vi "Teleop.vi"(10 "Match Info":T1={"Autonomous Elapsed Seconds"=0.0, "TeleOp Elapsed Seconds"=0.0, "Disabled Elapsed Seconds"=0.0, "Visited Autonomous"=FALSE, "Visited TeleOp"=FALSE, "Visited Disabled"=FALSE, "Autonomous Settings"={"Autonomous Style"=enum."Independent", "VI Refnum"=refnum}}, 11 "Call Context":T2) -> ()   [LabVIEW 2015]
doc: "This VI is called for each TeleOp packet received from the DS where the robot is not disabled. It is often used to read from the joysticks and update I/O or to update setpoints for timed control loops. It should complete and return within 20 milliseconds or it may miss DS packets."
uses:
  <vilib>/Rock Robotics/WPI/DriverStation/WPI_DriverStationDerivedRobotMode.ctl
  <vilib>/Rock Robotics/WPI/DriverStation/WPI_DriverStationMatch Info.ctl
  <vilib>/Rock Robotics/WPI/Utilities/WPI_GetSetVariantRefNum.vi
  <vilib>/Rock Robotics/Network Tables/SD Write Numeric Array.vi
  <vilib>/Rock Robotics/Network Tables/SD Write Boolean Array.vi
  Robot Global Data.vi
  <vilib>/Rock Robotics/WPI/RobotDrive/WPI_RobotDriveMecanumDrive_Cartesian.vi
  SimpleGyro/SimpleGyro.lvlib
panel:
  out "Angle":dbl
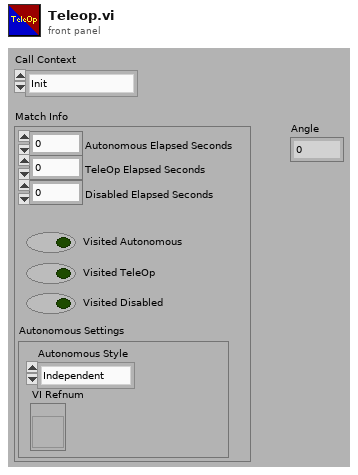
[diagram p1: front panel]
types:
  T1 = typedef "WPI_DriverStationMatch Info.ctl" = cluster{"Autonomous Elapsed Seconds":dbl, "TeleOp Elapsed Seconds":dbl, "Disabled Elapsed Seconds":dbl, "Visited Autonomous":bool, "Visited TeleOp":bool, "Visited Disabled":bool, "Autonomous Settings":cluster{"Autonomous Style":enum16{"Iterative", "Independent"}, "VI Refnum":refnum<vi>}}
  T2 = typedef "WPI_DriverStationDerivedRobotMode.ctl" = enum16{"Init", "Execute", "Stop"}
  T3 = typedef "WPI_JoystickDevRef.ctl" = cluster{"Device":T4}
  T4 = typedef "WPI_JoystickDeviceEnum.ctl" = enum16{"USB 0", "USB 1", "USB 2", "USB 3", "USB 4", "USB 5"}
  T5 = typedef "WPI_RobotDriveDevRef.ctl" = cluster{"DevStatus":errorcluster, "Motors[]":T6[], "Square Inputs":bool, "Max Output":dbl}
  T6 = typedef "WPI_MotorControlDeviceRef.ctl" = cluster{"DeviceStatus":errorcluster, "Type":T7, "PWM":cluster{"PWM Channel":T8, "DeadBand":T9}, "CAN":cluster{"Device Number":u8, "Control Mode":T10, "Semaphore":T11, "Max Vout":dbl, "TalonSRX Control Mode":T12}, "Invert":bool, "TransformRef":T13, "InvTransformRef":T13}
  T7 = typedef "WPI_MotorControlType.ctl" = enum16{"PWM", "CAN", "CANTalonSRX"}
  T8 = typedef "FPGA_DIOPWMChannel.ctl" = enum8{"PWM 0", "PWM 1", "PWM 2", "PWM 3", "PWM 4", "PWM 5", "PWM 6", "PWM 7", "PWM 8", "PWM 9", "PWM MXP 0", "PWM MXP 1", "PWM MXP 2", "PWM MXP 3", "PWM MXP 4", "PWM MXP 5", "PWM MXP 6", "PWM MXP 7", "PWM MXP 8", "PWM MXP 9", "Invalid"}
  T9 = typedef "WPI_PWMDeadband.ctl" = cluster{"Name":string, "maxPositivePwm":i32, "minPositivePwm":i32, "centerPwm":i32, "maxNegativePwm":i32, "minNegativePwm":i32, "angularRange":u16}
  T10 = typedef "WPI_CANJaguar_ControlMode.ctl" = enum8{"Percent VBus", "Current", "Speed", "Position", "Voltage"}
  T11 = typedef "Semaphore RefNum" = refnum<k1>
  T12 = typedef "WPI_CANTalonSRX_APIControlMode.ctl" = enum8{"Percent VBus", "Speed", "Position", "Slave", "Unchanged / Invalid"}
  T13 = typedef "WPI_PWMTransform_ConPane.ctl" = refnum<vi>
  T14 = typedef "SimpleGyro.lvlib/WPI_SimpleGyroDevRef.ctl" = cluster{"DevStatus":errorcluster, "Handle":i32, "SPI Bus":T15, "Device Found":bool, "Sample Rate":dbl}
  T15 = typedef "spi_bus.ctl" = enum16{"SPI On-Board, CS0", "SPI On-Board, CS1", "SPI On-Board, CS2", "SPI On-Board, CS3", "SPI MXP", "Invalid"}
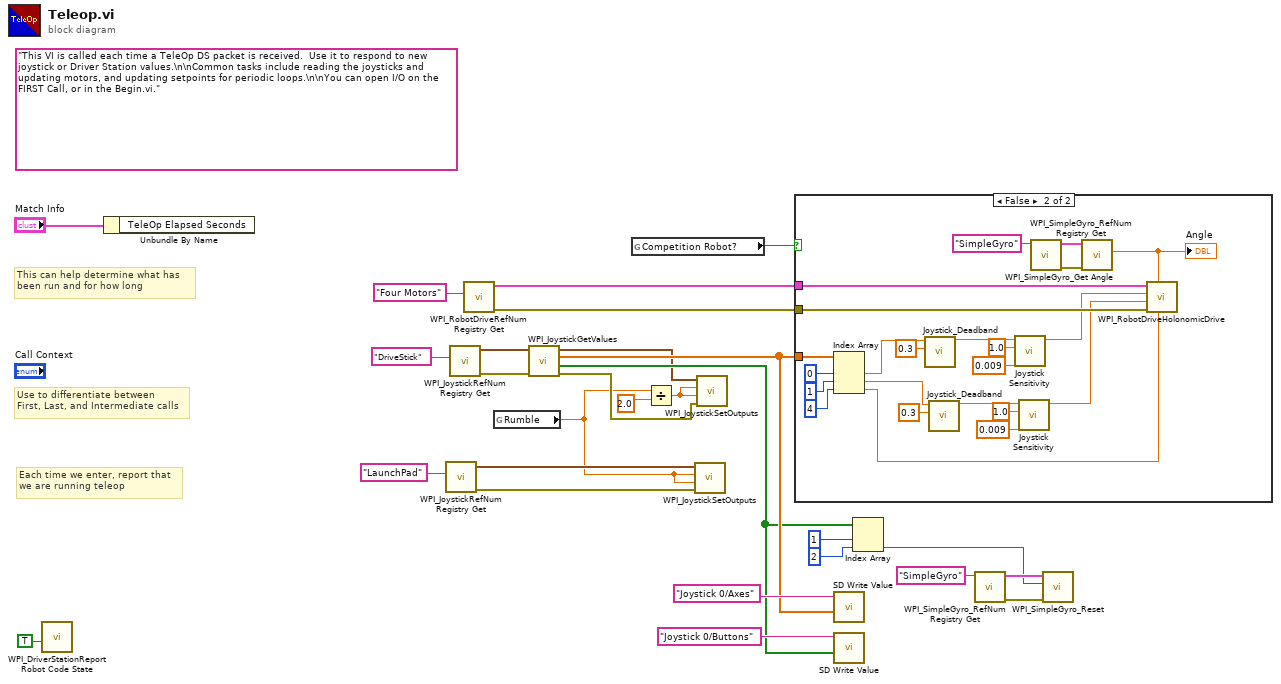
[diagram p0: block diagram]
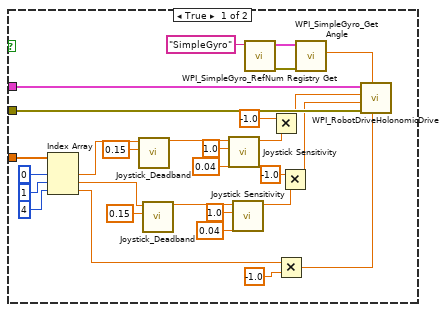
[diagram p2: hidden frame]
diagram:
  (unwired) "This VI is called each time a TeleOp DS packet is received.  Use it to respond to new joystick or Driver Station values.\n\nCommon tasks include reading the joysticks and updating motors, and updating setpoints for periodic loops.\n\nYou can open I/O on the FIRST Call, or in the Begin.vi."
  # "Each time we enter, report that\nwe are running teleop"
  # "Use to differentiate between\nFirst, Last, and Intermediate calls"
  # "This can help determine what has\nbeen run and for how long"
  n1 = call <vilib>:"WPI_DriverStationReport Robot Code State.vi"("TeleOp"=TRUE ("Autonomous")) -> ()  [unwired: 10 in, 1 out]
  n2 = Unbundle By Name("Match Info") -> ()  [unwired: 1 out]
  n3 = call <vilib>:"WPI_JoystickRefNum Registry Get.vi"("refnum name"="LaunchPad") -> ("error out"=w8:errorcluster, "JoystickDevRef"=w7:T3)  [unwired: 9 in]
  n4 = call <vilib>:"WPI_JoystickRefNum Registry Get.vi"("refnum name"="DriveStick") -> ("error out"=w19:errorcluster, "JoystickDevRef"=w21:T3)  [unwired: 9 in]
  n5 = call <vilib>:"WPI_RobotDriveRefNum Registry Get.vi"("refnum name"="Four Motors") -> ("error out"=w20:errorcluster, "RobotDriveDevRef"=w17:T5)  [unwired: 1 in, 8 out]
  n6 = global read "Robot Global Data.vi" "Rumble"() -> (w2:dbl)
  n7 = call <vilib>:"WPI_JoystickGetValues.vi"("error in (no error)"=w19, "JoystickDevRef"=w21) -> ("error out"=w10:errorcluster, "Buttons"=w22:bool[], "Axes"=w23:dbl[], "JoystickDevRef"=w11:T3)  [unwired: 5 in, 1 out]
  n8 = global read "Robot Global Data.vi" "Competition Robot?"() -> (w1:bool)
  n9 = Divide(x=w2, y=2.0) -> (x/y=w12:dbl)
  n10 = call <vilib>:"WPI_JoystickSetOutputs.vi"("error in (no error)"=w8, "Right Rumble"=w2, "Left Rumble"=w2, "JoystickDevRef"=w7) -> ()  [unwired: 6 in, 2 out]
  n11 = call <vilib>:"WPI_JoystickSetOutputs.vi"("error in (no error)"=w10, "Right Rumble"=w12, "Left Rumble"=w12, "JoystickDevRef"=w11) -> ()  [unwired: 6 in, 2 out]
  n12 = case shown="False" w1 {
    tunnel: w23 -> [w56 w79]
    tunnel: w20 -> [w55 w78]
    tunnel: w17 -> [w51 w74]
    frame True {
      n13 = Index Array(array=w56, index #1=0 ("index"), index #2=1 ("index"), index #3=4 ("index")) -> (element #1=w38:dbl, element #2=w43:dbl, element #3=w36:dbl)
      n14 = call "Joystick_Deadband.vi"("band"=0.15, "in"=w38) -> ("out"=w41:dbl)  [unwired: 9 in]
      n15 = call "Joystick_Deadband.vi"("band"=0.15, "in"=w43) -> ("out"=w46:dbl)  [unwired: 9 in]
      n16 = call "Joystick Sensitivity.vi"("B"=0.04, "A"=1.0, "X"=w41) -> ("Y"=w33:dbl)  [unwired: 8 in]
      n17 = call "Joystick Sensitivity.vi"("B"=0.04, "A"=1.0, "X"=w46) -> ("Y"=w32:dbl)  [unwired: 8 in]
      n18 = call "WPI_SimpleGyro_RefNum Registry Get.vi"("refnum name"="SimpleGyro") -> ("error out"=w47:errorcluster, "SimpleGyroDevRef"=w49:T14)  [unwired: 9 in]
      n19 = Multiply(x=-1.0, y=w33) -> (x*y=w31:dbl)
      n20 = Multiply(x=w36, y=-1.0) -> (x*y=w35:dbl)
      n21 = Multiply(x=-1.0, y=w32) -> (x*y=w29:dbl)
      n22 = call "WPI_SimpleGyro_Get Angle.vi"("error in"=w47, "SimpleGyroDevRef"=w49) -> ("Angle"=w50:dbl)  [unwired: 7 in, 2 out]
      n23 = call-poly <vilib>:"WPI_RobotDriveHolonomicDrive.vi"("Rotation"=w35, "Gyro Angle"=w50, "error in (no error)"=w55, "Y"=w29, "X"=w31, "RobotDriveDevRef"=w51) -> ()  [unwired: 3 in, 3 out]
    }
    frame False {
      n24 = Index Array(array=w79, index #1=0 ("index"), index #2=1 ("index"), index #3=4 ("index")) -> (element #1=w61:dbl, element #2=w66:dbl, element #3=w59:dbl)
      n25 = call "Joystick_Deadband.vi"("band"=0.3, "in"=w61) -> ("out"=w64:dbl)  [unwired: 9 in]
      n26 = call "Joystick_Deadband.vi"("band"=0.3, "in"=w66) -> ("out"=w69:dbl)  [unwired: 9 in]
      n27 = call "Joystick Sensitivity.vi"("B"=0.009, "A"=1.0, "X"=w64) -> ("Y"=w57:dbl)  [unwired: 8 in]
      n28 = call "Joystick Sensitivity.vi"("B"=0.009, "A"=1.0, "X"=w69) -> ("Y"=w58:dbl)  [unwired: 8 in]
      n29 = call "WPI_SimpleGyro_RefNum Registry Get.vi"("refnum name"="SimpleGyro") -> ("error out"=w70:errorcluster, "SimpleGyroDevRef"=w72:T14)  [unwired: 9 in]
      n30 = call "WPI_SimpleGyro_Get Angle.vi"("error in"=w70, "SimpleGyroDevRef"=w72) -> ("Angle"=w73:dbl)  [unwired: 7 in, 2 out]
      "Angle" <- w73
      n31 = call-poly <vilib>:"WPI_RobotDriveHolonomicDrive.vi"("Rotation"=w59, "Gyro Angle"=w73, "error in (no error)"=w78, "Y"=w58, "X"=w57, "RobotDriveDevRef"=w74) -> ()  [unwired: 3 in, 3 out]
    }
  }
  n32 = call-poly <vilib>:"SD Write Value.vi"("Numeric Array"=w23, "Name"="Joystick 0/Axes") -> ()  [unwired: 8 in, 2 out]
  n33 = call-poly <vilib>:"SD Write Value.vi"("Boolean Array"=w22, "Name"="Joystick 0/Buttons") -> ()  [unwired: 8 in, 2 out]
  n34 = Index Array(array=w22, index #1=1 ("index"), index #2=2 ("index")) -> (element #2=w3:bool)  [unwired: 1 out]
  n35 = call "WPI_SimpleGyro_RefNum Registry Get.vi"("refnum name"="SimpleGyro") -> ("error out"=w4:errorcluster, "SimpleGyroDevRef"=w5:T14)  [unwired: 9 in]
  n36 = call "WPI_SimpleGyro_Reset.vi"("error in"=w4, "Reset? (T)"=w3, "SimpleGyroDevRef"=w5) -> ()  [unwired: 7 in, 2 out]
